vi "Case Structures.vi"() -> ()   [LabVIEW 2019]
panel:
  in  "Choose Inifinity":i16
  in  "Choose B":bool
  out "Chosen":dbl
  in  "Choose A":bool
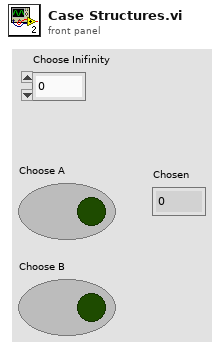
[diagram p1: front panel]
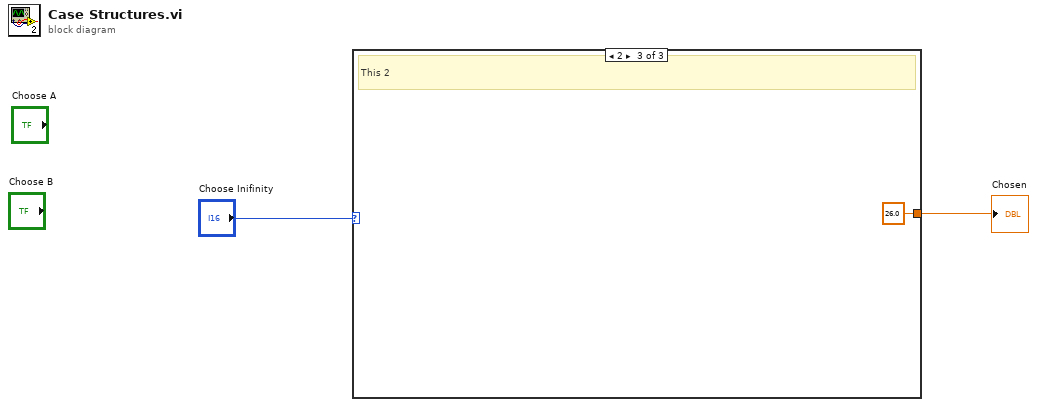
[diagram p0: block diagram]
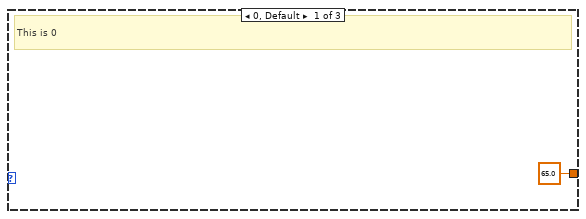
[diagram p2: hidden frame]
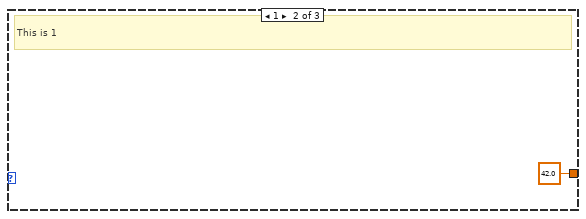
[diagram p3: hidden frame]
diagram:
  n1 = case shown="2" "Choose Inifinity" {
    tunnel: [65.0 42.0 26.0] -> w2
    frame 0, Default {
      # "This is 0"
    }
    frame 1 {
      # "This is 1"
    }
    frame 2 {
      # "This 2"
    }
  }
  "Chosen" <- w2
